vi "CSTK_BuildApplication Manager.vi"   [LabVIEW 2015]
uses:
  Library/BuildApplication Manager/CSTK_BuildApplication_Manager.lvlib
panel:
  # "BuildApplication Manager"
types:
  T1 = enum32{"Invalid", "Standard", "Closed", "Hidden", "Minimized", "Maximized"}
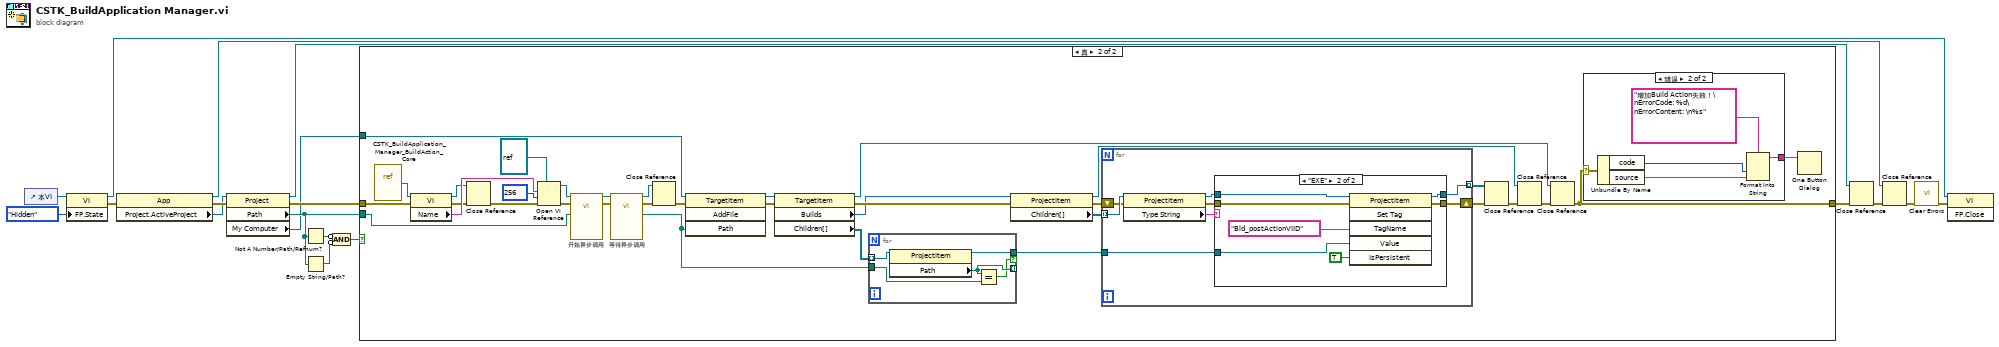
[diagram p0: block diagram]
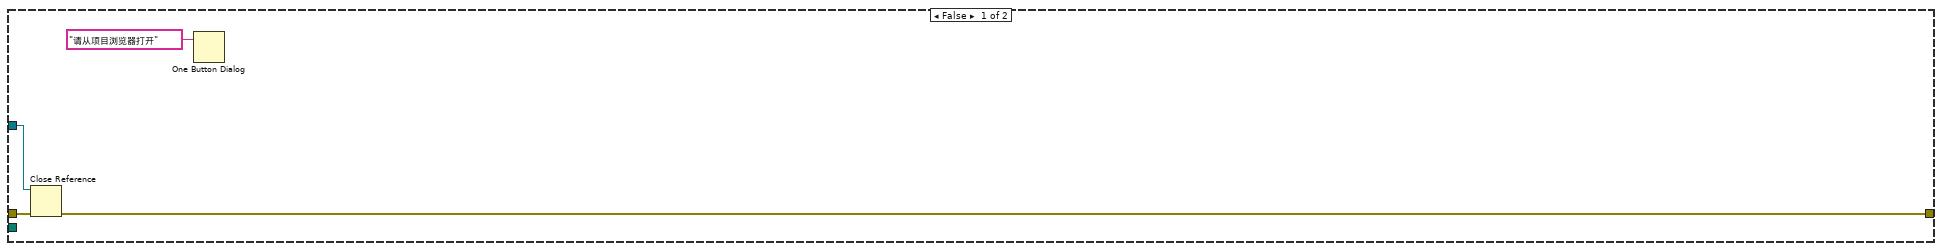
[diagram p2: hidden frame]
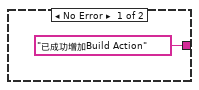
[diagram p3: hidden frame]
diagram:
  n1 = control-ref of="本VI"() -> (w18:refnum<vi>)
  n2 = property class="VI"(reference=w18, "FP.State"=T1."Hidden" ("前面板窗口:状态")) -> (reference out=w16:refnum<vi>, error out=w13:errorcluster)  [unwired: 1 in]
  n3 = property class="App"(error in=w13) -> (reference out=w4:refnum<vi>, error out=w15:errorcluster, "Project.ActiveProject"=w14:refnum<vi>)  [unwired: 1 in]
  n4 = property class="Project"(reference=w14, error in=w15) -> (reference out=w5:refnum<vi>, error out=w12:errorcluster, "Path"=w8:path, "My Computer"=w7:refnum<vi>)
  n5 = Not A Number/Path/Refnum?(number/path/refnum=w8) -> (NaN/Path/Refnum?=w10:bool)
  n6 = Empty String/Path?(string/path=w8) -> (empty?=w11:bool)
  n7 = Compound Arithmetic op=AND ("复合运算")(invert w10, invert w11) -> (w9:bool)
  n8 = case shown="真" w9 {
    tunnel: [w20 w24] -> w3
    tunnel: w12 -> [w21 w50]
    tunnel: w8 -> [_ w49]
    tunnel: w7 -> [w22 w43]
    frame False {
      n9 = Close Reference(reference=w22, error in (no error)=w21) -> (error out=w20:errorcluster)
      n10 = One Button Dialog(message="请从项目浏览器打开" ("消息")) -> ()  [unwired: 1 in, 1 out]
    }
    frame True {
      n11 = vi-ref "CSTK_BuildApplication_Manager_BuildAction_Core.vi"() -> (w55:refnum<vi>)
      n12 = property class="VI"(reference=w55, error in=w50) -> (reference out=w31:refnum<vi>, error out=w33:errorcluster, "Name"=w56:string)
      n13 = Close Reference(reference=w31, error in (no error)=w33) -> (error out=w32:errorcluster)
      n14 = Open VI Reference(type specifier VI Refnum (for type only)=refnum<vi> refnum ("类型说明符VI引用句柄（仅用于类型）"), vi path=w56, options=256 ("选项"), error in (no error)=w32) -> (vi reference=w51:refnum<vi>, error out=w53:errorcluster)  [unwired: 2 in]
      n15 = call-by-ref "开始异步调用"(reference=w51, error in=w53, "项目路径"=w49) -> (reference out=w48:refnum<vi>, error out=w47:errorcluster)  [unwired: 9 in, 2 out]
      n16 = call-by-ref "等待异步调用"(reference=w48, error in=w47) -> (reference out=w46:refnum<vi>, error out=w45:errorcluster, "SavePath"=w39:path)  [unwired: 10 in, 1 out]
      n17 = Close Reference(reference=w46, error in (no error)=w45) -> (error out=w44:errorcluster)
      n18 = invoke class="TargetItem" method="AddFile"(reference=w43, error in=w44, "Path"=w39) -> (reference out=w42:refnum<vi>, error out=w41:errorcluster)  [unwired: 1 in, 2 out]
      n19 = property class="TargetItem"(reference=w42, error in=w41) -> (reference out=w25:refnum<vi>, error out=w38:errorcluster, "Builds"=w37:refnum<vi>, "Children[]"=w40:refnum<vi>[])
      n20 = for {
        tunnel: w40 -> [w84] mode=indexing
        tunnel: [w83] -> _ mode=indexing
        tunnel: w39 -> [w82]
        tunnel: [w81] -> w35 if=w80
        n21 = property class="ProjectItem"(reference=w84) -> (reference out=w81:refnum<vi>, "Path"=w83:path)  [unwired: 1 in, 1 out]
        n22 = Equal?(x=w83, y=w82) -> (x = y?=w80:bool)
      }
      n23 = property class="ProjectItem"(reference=w37, error in=w38) -> (reference out=w28:refnum<vi>, error out=w34:errorcluster, "Children[]"=w36:refnum<vi>[])
      n24 = for {
        tunnel: w36 -> [w70] mode=indexing
        tunnel: w35 -> [w67]
        shift-right: [w64] -> w30
        shift-left: w34 -> [w66]
        tunnel: [w63] -> w29 mode=indexing
        n25 = property class="ProjectItem"(reference=w70, error in=w66) -> (reference out=w69:refnum<vi>, error out=w65:errorcluster, "Type String"=w68:string)
        n26 = case shown="\"EXE\"" w68 {
          tunnel: w69 -> [w71 w79]
          tunnel: w67 -> [_ w76]
          tunnel: w65 -> [w72 w75]
          tunnel: [w72 w74] -> w64
          tunnel: [w71 w73] -> w63
          frame Default {
          }
          frame "EXE" {
            n27 = invoke class="ProjectItem" method="Set Tag"(reference=w79, error in=w75, "TagName"="Bld_postActionVIID" ("标识符名"), "Value"=w76, "IsPersistent"=TRUE ("持续")) -> (reference out=w73:refnum<vi>, error out=w74:errorcluster)  [unwired: 1 in, 4 out]
          }
        }
      }
      n28 = Close Reference(reference=w29, error in (no error)=w30) -> (error out=w27:errorcluster)
      n29 = Close Reference(reference=w28, error in (no error)=w27) -> (error out=w26:errorcluster)
      n30 = Close Reference(reference=w25, error in (no error)=w26) -> (error out=w24:errorcluster)
      n31 = case shown="错误" w24 {
        selector: w24 -> [_ w60]
        tunnel: ["已成功增加Build Action" w61] -> w23
        frame No Error {
        }
        frame Error {
          n32 = Unbundle By Name(w60) -> ("code"=w59:i32, "source"=w58:string)
          n33 = Format Into String(format string="增加Build Action失败！\nErrorCode: %d\nErrorContent: \n%s" ("格式字符串"), w59, w58) -> (resulting string=w61:string)  [unwired: 2 in, 1 out]
        }
      }
      n34 = One Button Dialog(message=w23) -> ()  [unwired: 1 in, 1 out]
    }
  }
  n35 = Close Reference(reference=w5, error in (no error)=w3) -> (error out=w6:errorcluster)
  n36 = Close Reference(reference=w4, error in (no error)=w6) -> (error out=w1:errorcluster)
  n37 = call <vilib>:"Clear Errors.vi"("error in (no error)"=w1) -> ("error out"=w2:errorcluster)  [unwired: 5 in, 1 out]
  n38 = invoke class="VI" method="FP.Close"(reference=w16, error in=w2) -> ()  [unwired: 1 in, 3 out]
